vi "Get New Level.vi"(8 "error in (no error)":errorcluster, 11 "Water Level in":refnum<class "Water Level.lvclass">) -> (0 "error out":errorcluster, 2 "Level":dbl, 3 "Water Level out":refnum<class "Water Level.lvclass">)   [LabVIEW 2012, in "Water Level.lvclass"]
uses:
  Water Level.lvclass
  Simulation/Simulation Data_Global.vi
  Simulation/Simulation.lvlib
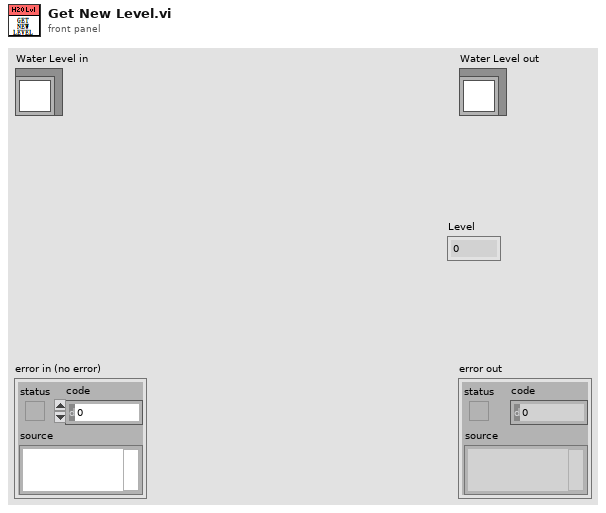
[diagram p1: front panel]
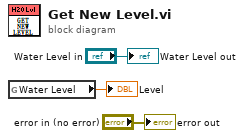
[diagram p0: block diagram]
diagram:
  n1 = global read "Simulation Data_Global.vi" "Water Level"() -> (→"Level":dbl)
  "error out" <- "error in (no error)"
  "Water Level out" <- "Water Level in"
